vi "Untitled 1.vi"() -> ()   [LabVIEW 2015]
uses:
  <instrlib>/Agilent 34401/Public/Data/Read (Multiple Points).vi
  <instrlib>/Agilent 34401/Agilent 34401.lvlib
panel:
  out "Waveform Graph":waveform(dbl)(graph)
  in  "stop":bool
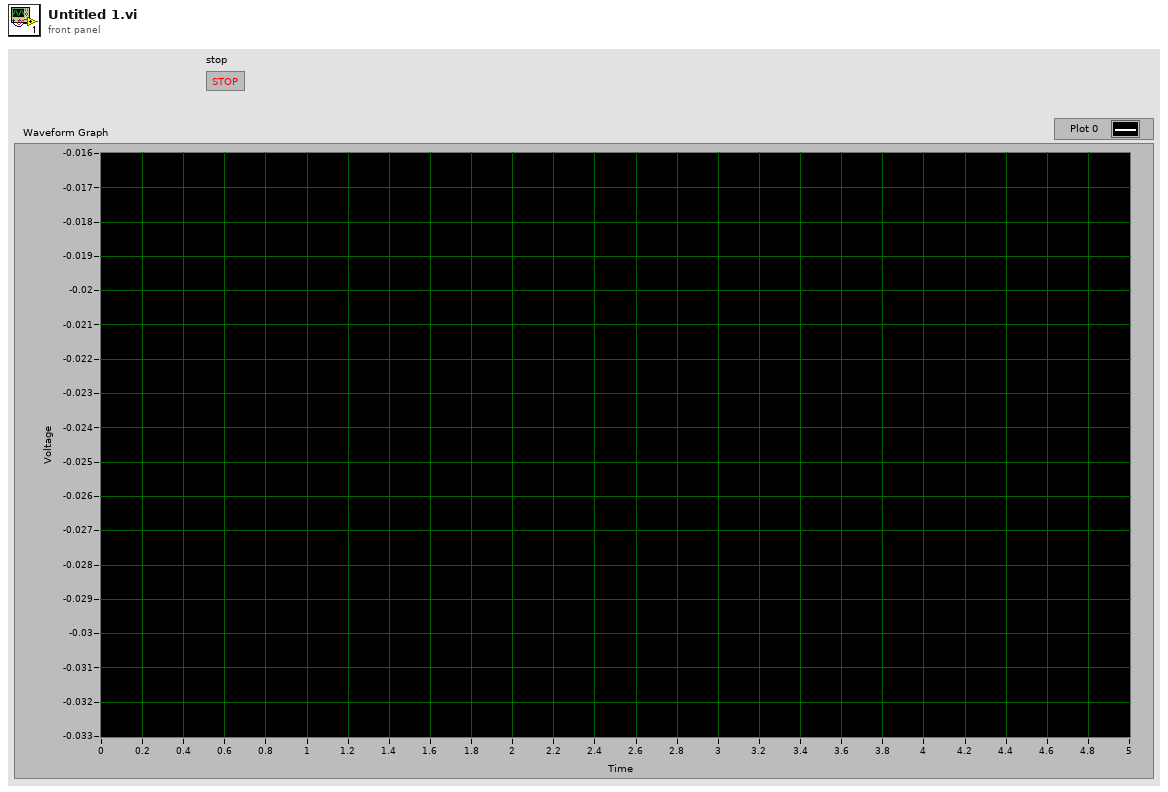
[diagram p1: front panel]
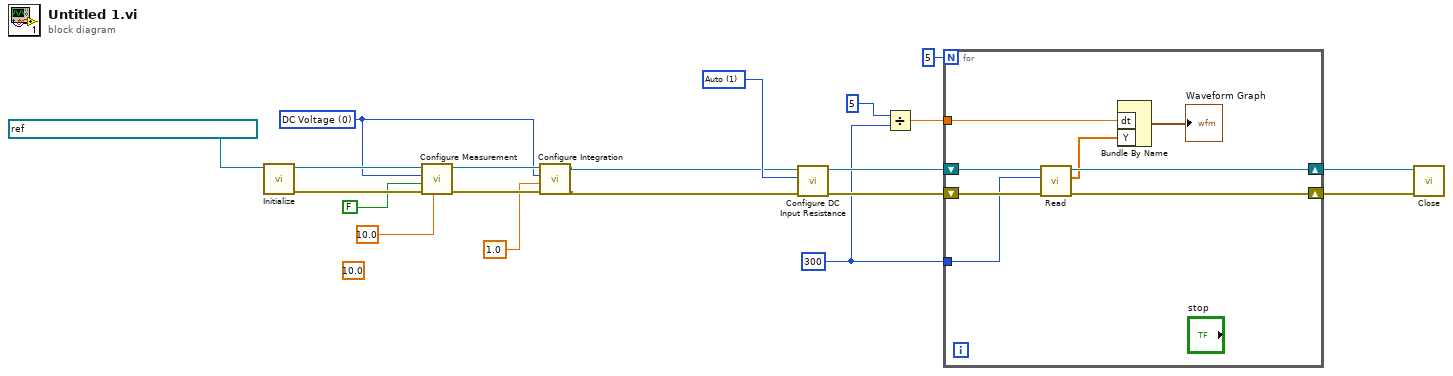
[diagram p0: block diagram]
diagram:
  w7 = u16 1 items=["Fixed", "Auto"] ("DC Input Resistance Mode (0: Fixed)")
  w11 = 1.0 items=["0.001"=0.001, "0.002"=0.002, "0.006"=0.006, "0.02"=0.02, "0.06"=0.06, "0.2"=0.2, "1"=1.0, "10"=10.0, "100"=100.0] ("Integration Time (1 PLCs)")
  (unwired) 10.0 ("Manual Range (1.00)")
  w2 = 300 ("Sample Count (1)")
  w12 = u16 0 items=["DC Voltage", "AC Voltage", "2 - Wire Resistance", "4 - Wire Resistance", "DC Current", "AC Current", "Frequency", "Period", "Continuity", "Diode Checking", "VDC:VDC Ratio", "Temperature", "Capacitance"] ("Function (0: DC Voltage)")
  n1 = call <instrlib>:"Initialize.vi"("VISA resource name"=refnum<visa-resource-name> "USB0::0x0957::0x0A07::MY53002732::INSTR") -> ("error out"=w18:errorcluster, "VISA resource name out"=w19:refnum<visa-resource-name>)  [unwired: 9 in]
  n2 = call <instrlib>:"Configure Measurement.vi"("Manual Range (1.00)"=10.0, "error in (no error)"=w18, "Enable Auto Range (T: Enable)"=FALSE, "Function (0: DC Voltage)"=w12, "VISA resource name"=w19) -> ("error out"=w13:errorcluster, "VISA resource name out"=w14:refnum<visa-resource-name>)  [unwired: 5 in]
  n3 = call <instrlib>:"Configure Integration.vi"("error in (no error)"=w13, "Integration Time (1 PLCs)"=w11, "Function (0: DC Voltage)"=w12, "VISA resource name"=w14) -> ("error out"=w4:errorcluster, "VISA resource name out"=w5:refnum<visa-resource-name>)  [unwired: 6 in]
  n4 = call <instrlib>:"Configure DC Input Resistance.vi"("error in (no error)"=w4, "DC Input Resistance Mode (0: Fixed)"=w7, "VISA resource name"=w5) -> ("error out"=w9:errorcluster, "VISA resource name out"=w8:refnum<visa-resource-name>)  [unwired: 7 in]
  n5 = Divide(x=5, y=w2) -> (x/y=w3:dbl)
  n6 = for {
    N: 5 -> [_]
    shift-right: [w25] -> w16
    shift-left: w8 -> [w27]
    shift-right: [w26] -> w15
    shift-left: w9 -> [w28]
    tunnel: w2 -> [w24]
    tunnel: w3 -> [w22]
    n7 = call-poly <instrlib>:"Read.vi"("error in (no error)"=w28, "Sample Count (1)"=w24, "VISA resource name"=w27) -> ("error out"=w26:errorcluster, "Measurements"=w23:dbl[], "VISA resource name out"=w25:refnum<visa-resource-name>)  [unwired: 6 in]
    n8 = Bundle By Name("dt"=w22, "Y"=w23) -> (→"Waveform Graph":waveform(dbl))  [unwired: 1 in]
  }
  n9 = call <instrlib>:"Close.vi"("error in (no error)"=w15, "VISA resource name"=w16) -> ()  [unwired: 9 in, 1 out]
